vi "Graphics-Set Log Ticks.vi"(8 "Step":dbl=1.0, 9 "Base":dbl=2.0, 10 "Max":dbl, 11 "Min":dbl) -> (3 "Tick Vals":dbl[](array[numeric]))   [LabVIEW 2020]
uses:
  Math VIs/LinSpace (start-stop-step).vi
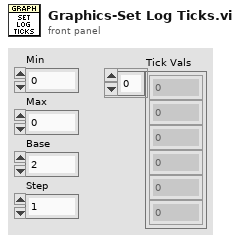
[diagram p1: front panel]
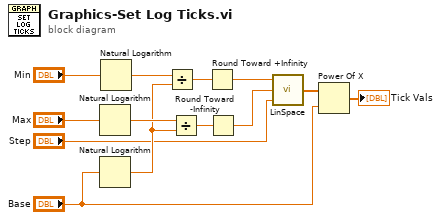
[diagram p0: block diagram]
diagram:
  n1 = Natural Logarithm(1:"Max") -> (0:w9:dbl)
  n2 = Natural Logarithm(1:"Base") -> (0:w8:dbl)
  n3 = Natural Logarithm(1:"Min") -> (0:w12:dbl)
  n4 = Divide(x=w12, y=w8) -> (x/y=w11:dbl)
  n5 = Divide(x=w9, y=w8) -> (x/y=w7:dbl)
  n6 = Round Toward +Infinity(x=w11) -> (ceil(x): smallest int >= x=w6:dbl)
  n7 = Round Toward -Infinity(1:w7) -> (0:w5:dbl)
  n8 = call-poly "LinSpace.vi"("Step"="Step", "Stop"=w5, "Start"=w6) -> ("Array"=w2:dbl[])  [unwired: 1 in, 1 out]
  n9 = Power Of X(1:"Base", 2:w2) -> (0:→"Tick Vals":dbl[])
